vi "Get Thread Configuration.vi"(8 "error in (no error)":errorcluster, 11 "Component Configuration in":refnum<class "UDP Configurations.lvclass">) -> (0 "error out":errorcluster, 2 "Thread Configuration":refnum<class "Configuration.lvclass">, 3 "Component Configuration out":refnum<class "UDP Configurations.lvclass">)   [LabVIEW 2023, in "UDP.lvlib" / "UDP Configurations.lvclass"]
uses:
  UDP Configurations.lvclass
  Users/Public/Documents/National Instruments/NI VeriStand 2023/Custom Devices/Data Sharing Framework/Linux_x64/DSF Core.lvlibp/Classes/Configuration/Configuration.lvclass
  Thread/UDP Thread Configuration.lvclass
  C:/Users/Public/Documents/National Instruments/NI VeriStand 2023/Custom Devices/Data Sharing Framework/Linux_x64/DSF Core.lvlibp/Classes/Configuration/Configuration.lvclass
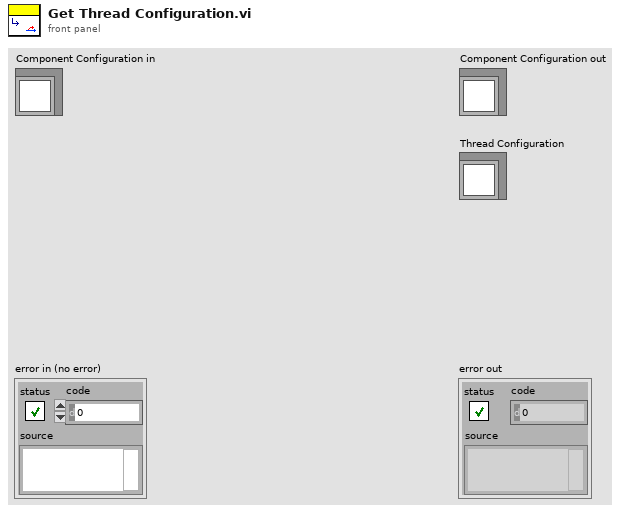
[diagram p1: front panel]
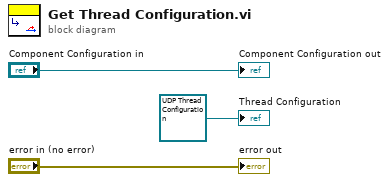
[diagram p0: block diagram]
diagram:
  "error out" <- "error in (no error)"
  "Component Configuration out" <- "Component Configuration in"
  "Thread Configuration" <- refnum<class "UDP Thread Configuration.lvclass"> refnum ("UDP Transceiver.lvlib:DSF UDP Thread Configuration")
